vi "Funnel Edit.vi"() -> ()   [LabVIEW 2019]
uses:
  Classes/Settings/Funnel Settings/Funnel Settings.lvclass/Funnel Settings.ctl
  Classes/Settings/ObjectSettings/ObjectSettings.lvclass/ObjectSettings.ctl
  typedefs/Schedule Types/Schedule--Constant.ctl
  Classes/Settings/Setting Database/Setting Database.lvclass
  Classes/Settings/Funnel Settings/Funnel Settings.lvclass
  C:/Users/Albro/Documents/GitHub/AFM-Lithography/lvsrc/Classes/Settings/ObjectSettings/ObjectSettings.lvclass
  Classes/Settings/Setting Database/Typedefs/PrivateEvents--Setting Database.SetDefaultFunnel.ctl
  Classes/Settings/Setting Database/Typedefs/PrivateEvents--Setting Database.CopyActiveFunnelToAll.ctl
  <vilib>/JKI/JKI SMO/SMO/SMO.lvclass
  Classes/Settings/Funnel Settings/Accessors/Write Bottom Segments.vi
  Classes/Settings/ObjectSettings/Accessors/Write Resistance.vi
  Classes/Settings/ObjectSettings/Accessors/Read Speed Settings.vi
  Classes/Settings/ObjectSettings/Accessors/Read Voltage Settings.vi
  Classes/Settings/ObjectSettings/Accessors/Write Enabled.vi
  Classes/Settings/ObjectSettings/Accessors/Write Voltage Schedule.vi
  Classes/Settings/ObjectSettings/Accessors/Write Speed Schedule.vi
  Classes/Settings/ObjectSettings/Accessors/Write Direction.vi
  Classes/Settings/Funnel Settings/Accessors/Write Smooth Segments.vi
  Classes/Settings/ObjectSettings/Accessors/Read Enabled.vi
  Classes/Settings/ObjectSettings/Accessors/Read Direction.vi
  Classes/Settings/Funnel Settings/Accessors/Read Smooth Segments.vi
  Classes/Settings/Funnel Settings/Accessors/Read Bottom Segments.vi
  Classes/Settings/ObjectSettings/Accessors/Read Speed Schedule.vi
  Classes/Settings/ObjectSettings/Accessors/Read Voltage Schedule.vi
  Classes/Settings/ObjectSettings/Accessors/Read Resistance.vi
  Classes/Settings/ObjectSettings/ObjectSettings.lvclass
panel:
  in  "Save Default":bool
  out "resources found?":bool
  in  "Speed Settings":bool
  in  "Voltage Settings":bool
  in  "Smooth Segments":dbl caption="Numeric 2"
  in  "Set Resistance":T1(ring) caption="Enum"
  in  "Copy to All":bool
  in  "Bottom Segments":dbl caption="Numeric 2"
  in  "Voltage (V)":dbl caption="Numeric 2"
  in  "Speed (um/s)":dbl caption="Numeric 2"
  in  "Voltage Schedule":u16(ring) caption="Ring" items=["Constant", "Ramp", "Fn. Generator", "Formula"]
  in  "Speed Schedule":u16(ring) caption="Ring" items=["Constant", "Ramp", "Fn. Generator", "Formula"]
  in  "Direction":u16(ring) caption="Ring" items=["Forward", "Backward"]
  in  "Enabled?":bool=TRUE
  in  "Index":i32=8
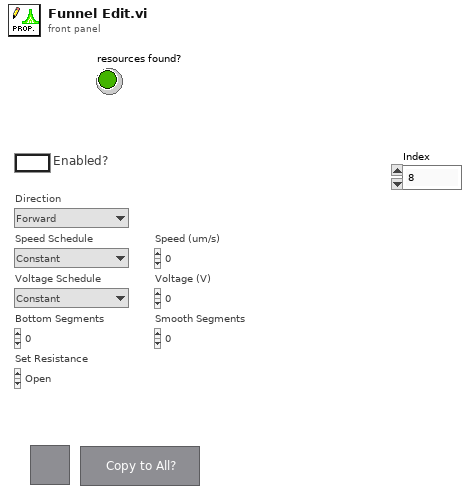
[diagram p1: front panel]
types:
  T1 = enum16{"Open", "Discharge Tip", "0 ohm", "100 kohm", "10 Mohm", "1 Gohm"}
  T2 = typedef "Schedule--Constant.ctl" = cluster{"Value":dbl}
  T3 = enum32{"invalid app kind", "Development System", "Run Time System", "Student Edition", "Embedded LabVIEW", "Evaluation", "Custom"}
  T4 = enum8{"Enabled", "Disabled", "Disabled and Grayed Out"}
  T5 = enum32{"Invalid", "Standard", "Closed", "Hidden", "Minimized", "Maximized"}
  T6 = typedef "Setting Database.lvclass/PrivateEvents--Setting Database.SetDefaultFunnel.ctl" = bool
  T7 = typedef "Setting Database.lvclass/PrivateEvents--Setting Database.CopyActiveFunnelToAll.ctl" = bool
  T8 = typedef "Setting Database.lvclass/PublicEvents--Setting Database.NewActiveFunnel.ctl" = refnum<class "Funnel Settings.lvclass">
  T9 = cluster{"Core":cluster{"Current VI Reference":refnum<vi>, "Close Panel on Exit?":bool}, "SettingDB":refnum<class "Setting Database.lvclass">, "Funnel Settings":refnum<class "Funnel Settings.lvclass">}
  T10 = cluster{"Current VI Reference":refnum<vi>, "Close Panel on Exit?":bool}
  T11 = typedef "Setting Database.lvclass/PublicEvents--Cluster.ctl" = cluster{"NewActivePath":refnum<user-event>, "PathsUpdated":refnum<user-event>, "RectanglesUpdated":refnum<user-event>, "NewActiveRectangle":refnum<user-event>, "NewActiveFunnel":refnum<user-event>, "FunnelsUpdated":refnum<user-event>, "NewActiveDot":refnum<user-event>, "DotsUpdated":refnum<user-event>}
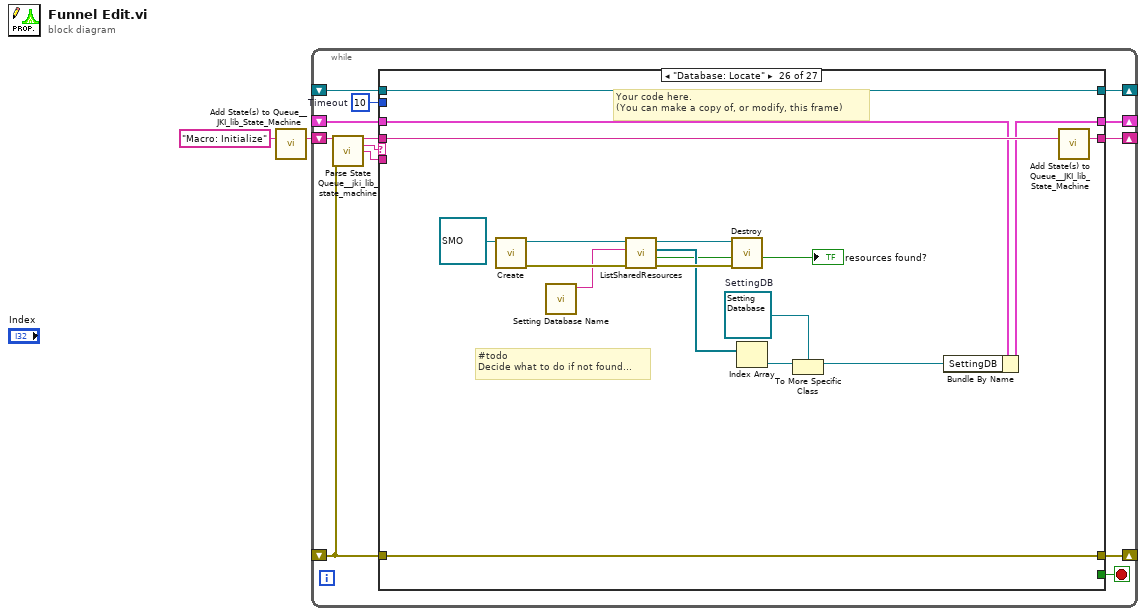
[diagram p0: block diagram]
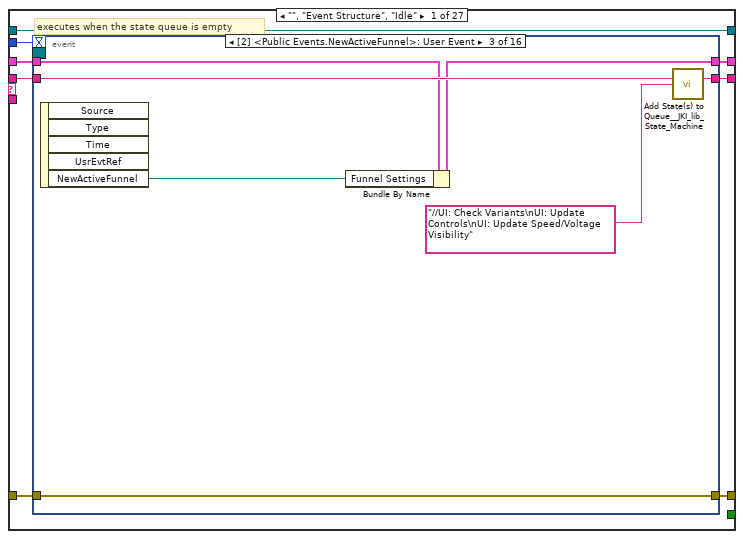
[diagram p2: hidden frame]
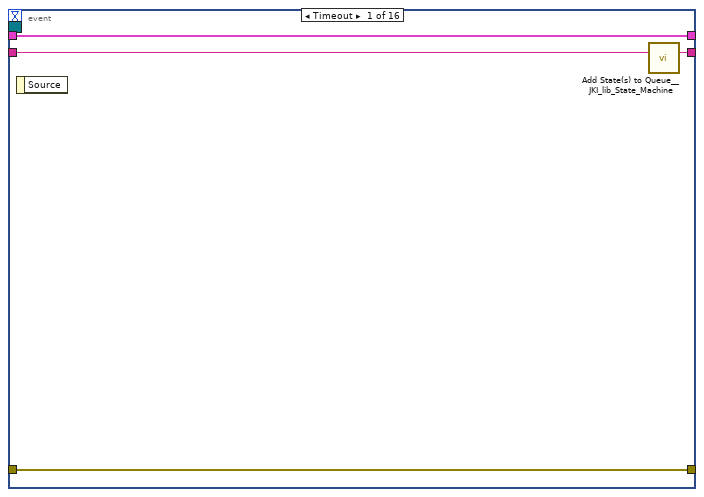
[diagram p3: hidden frame]
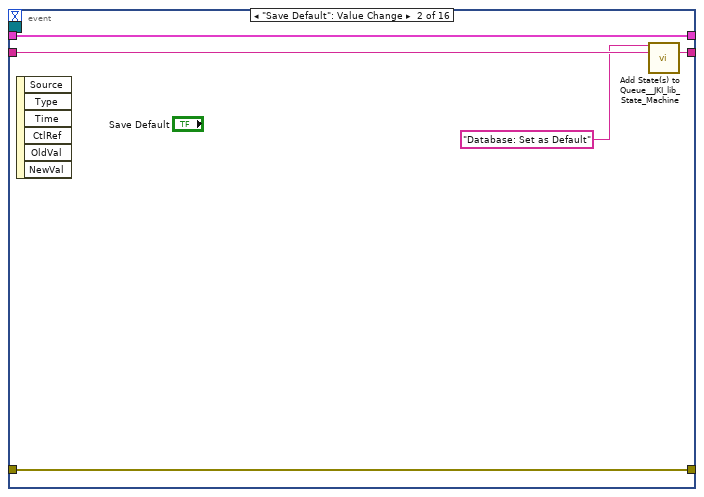
[diagram p4: hidden frame]
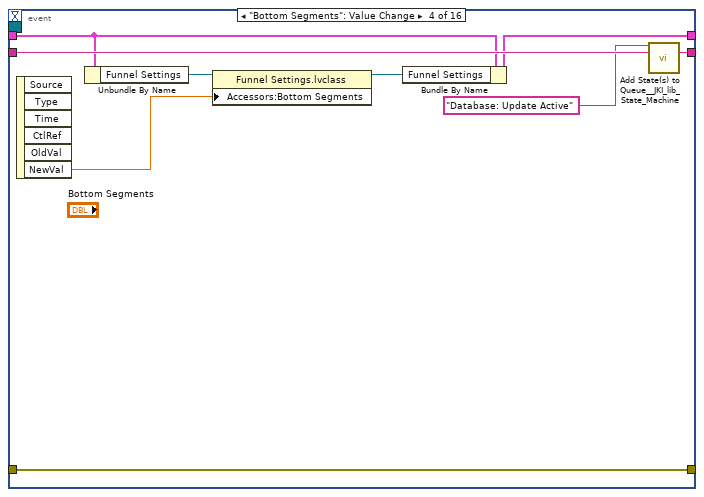
[diagram p5: hidden frame]
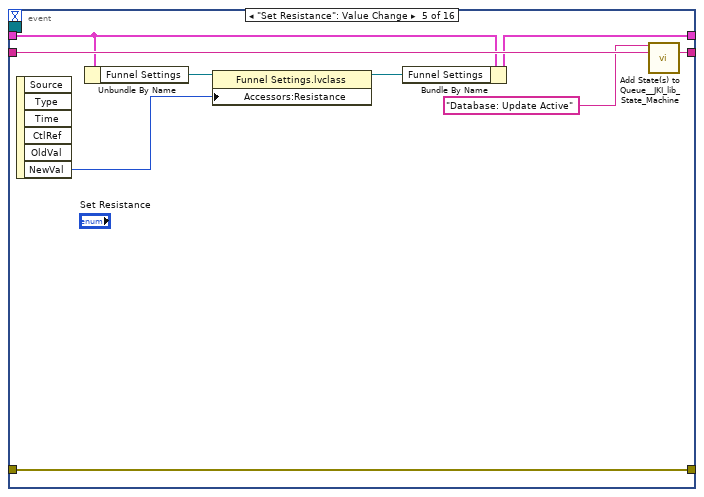
[diagram p6: hidden frame]
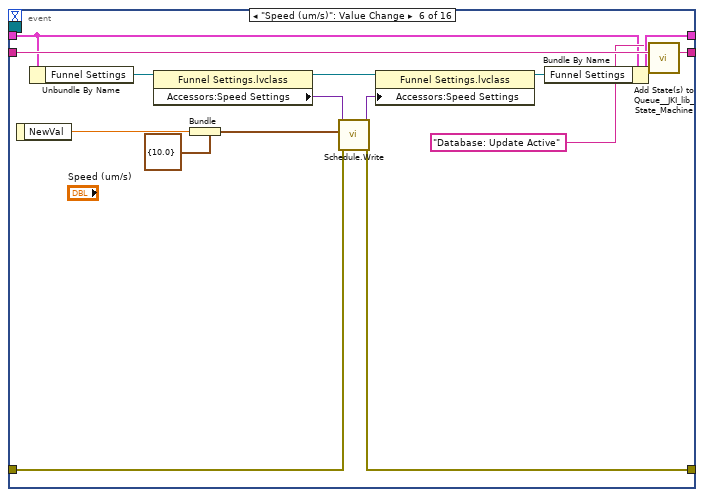
[diagram p7: hidden frame]
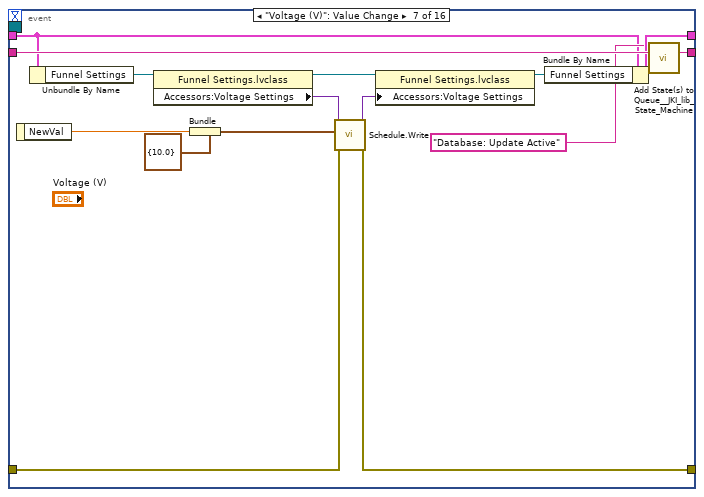
[diagram p8: hidden frame]
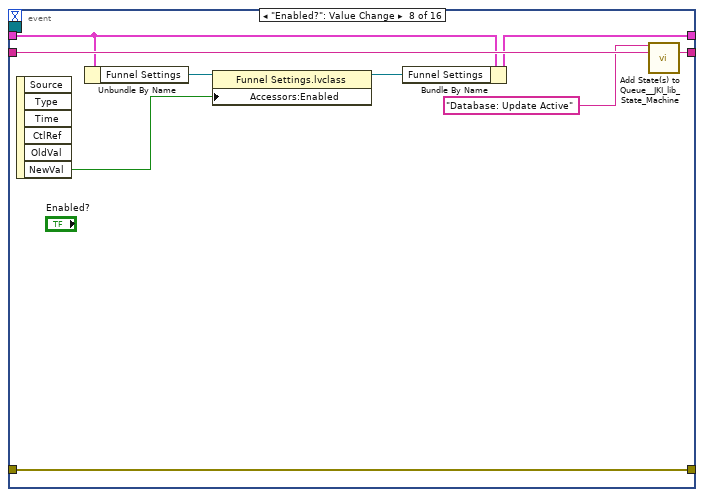
[diagram p9: hidden frame]
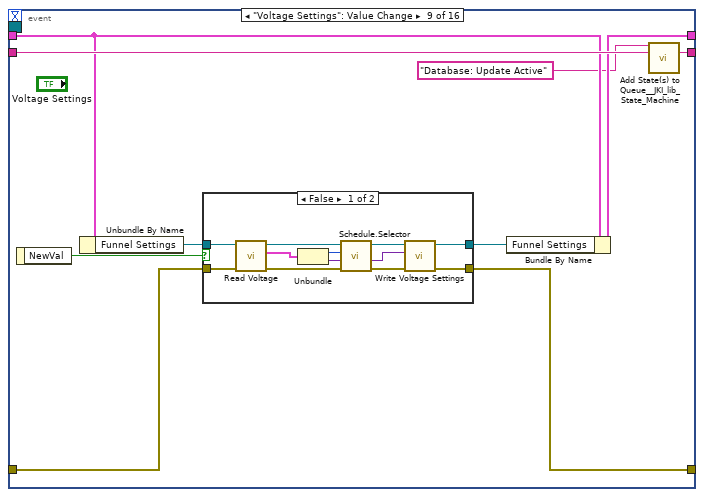
[diagram p10: hidden frame]
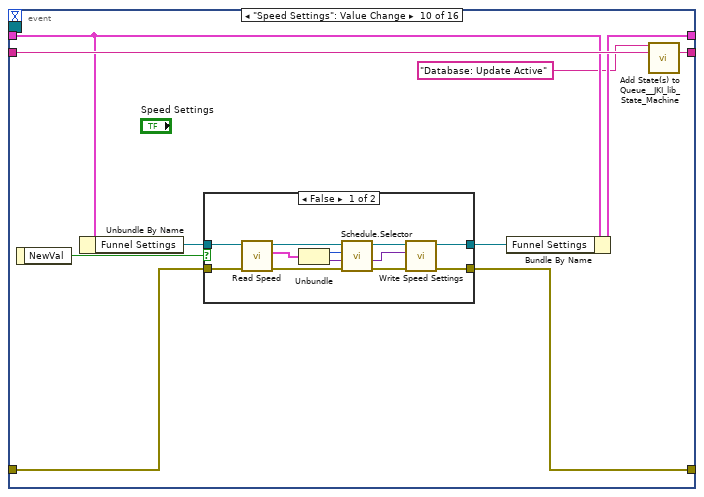
[diagram p12: hidden frame]
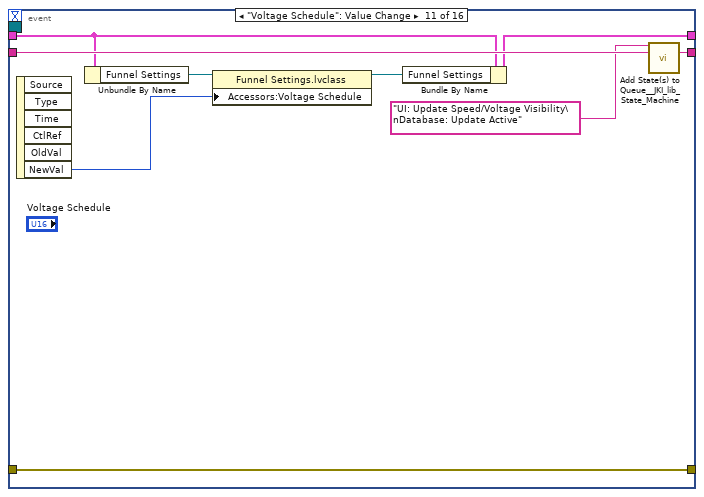
[diagram p14: hidden frame]
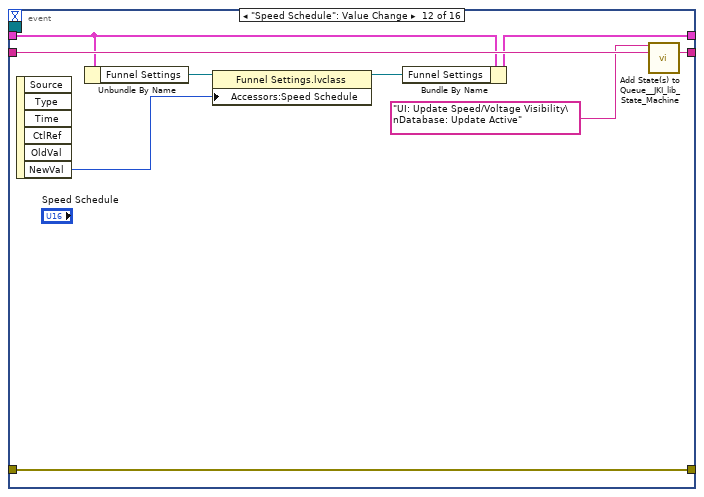
[diagram p15: hidden frame]
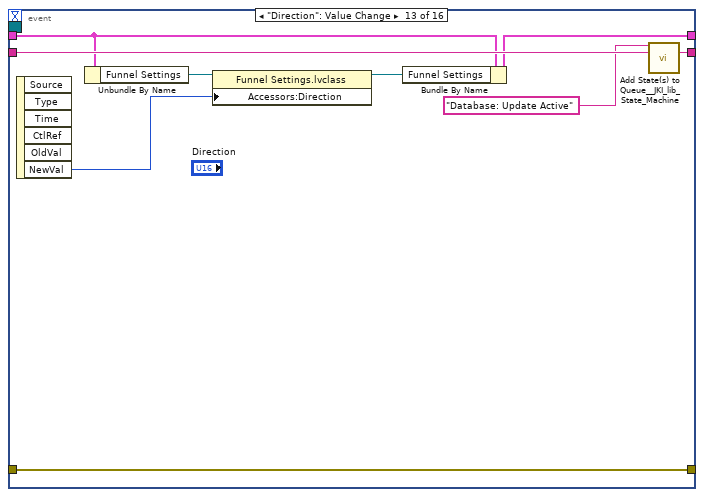
[diagram p16: hidden frame]
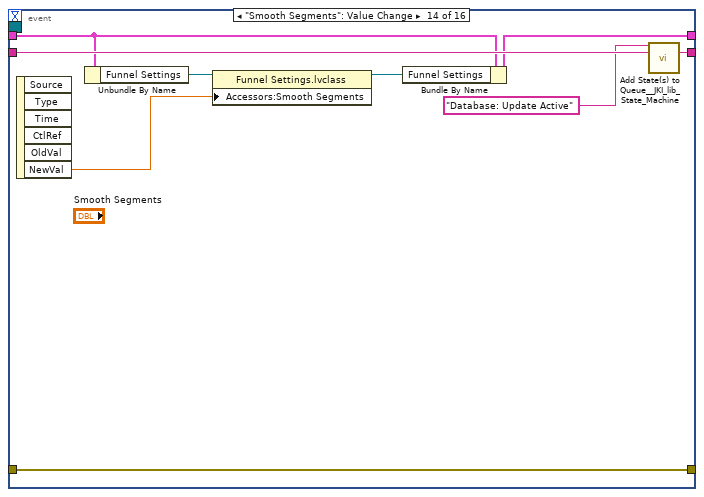
[diagram p17: hidden frame]
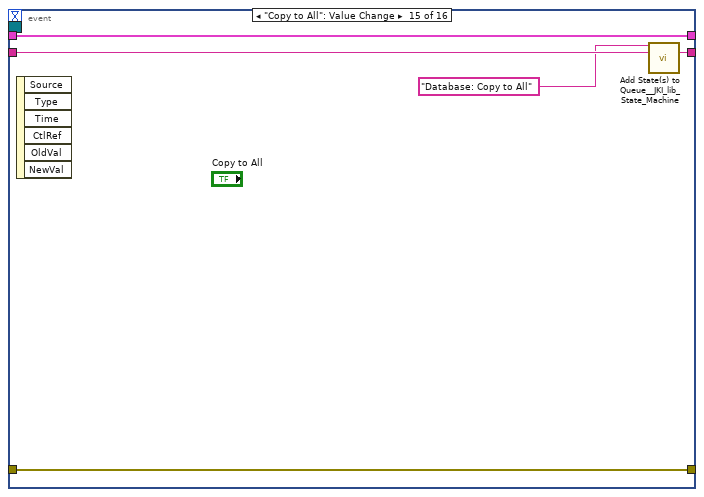
[diagram p18: hidden frame]
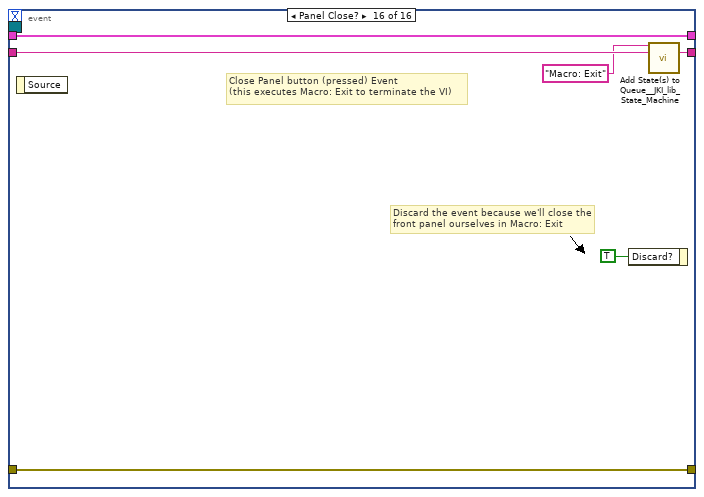
[diagram p19: hidden frame]
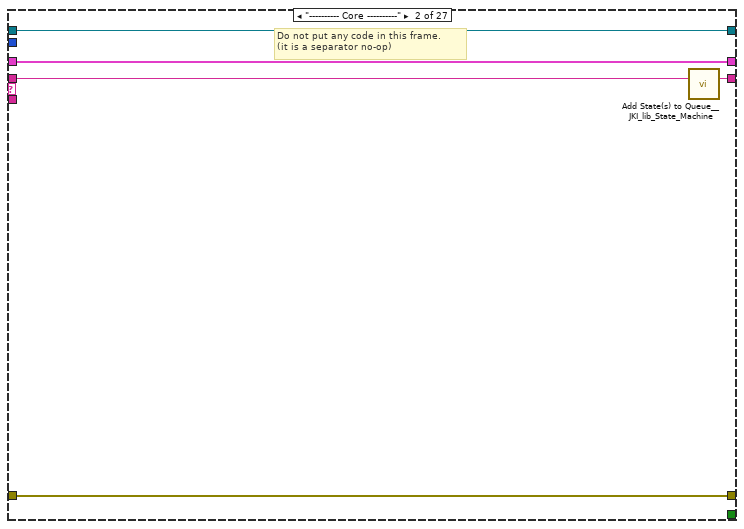
[diagram p20: hidden frame]
diagram:
  n1 = call <vilib>:"Add State(s) to Queue__JKI_lib_State_Machine.vi"("State(s) in (\"\")"="Macro: Initialize") -> ("States Out"=w2:string)  [unwired: 14 in]
  n2 = while "JKI - String-Based Queued State Machine (Basic) v1.0" {
    shift-right: [w8] -> _
    shift-left: _ -> [w7]
    shift-right: [w11] -> _
    shift-left: _ -> [w5]
    shift-right: [w10] -> _
    shift-left: w2 -> [w12]
    shift-right: [w4] -> _
    shift-left: _ -> [w3]
    stop <- w9 stop-if-true
    w6 = 10  # Timeout
    n3 = call <vilib>:"Parse State Queue__jki_lib_state_machine.vi"("State Queue"=w12, "Error In (no error)"=w5) -> ("Remaining States"=w14:string, "Current State"=w15:string, "Arguments"=w13:string)  [unwired: 11 in]
    n4 = case shown="\"Database: Locate\"" w15 {
      selector: w15 -> [_ _ w202 _ _ _ _ _ _ _ _ _ _ _ _ _ _ _ _ _ _ _ _ _ _ _ _]
      tunnel: w14 -> [w23 w196 w200 w221 w228 w234 w239 w247 w254 w259 w269 w275 w280 w288 w312 w327 w334 w353 w365 w392 w398 w409 w414 w424 w434 w451 w461]
      tunnel: w13 -> [_ _ _ _ _ _ _ _ _ _ _ _ _ _ _ _ w330 _ w360 _ _ _ _ _ _ _ _]
      tunnel: w7 -> [w21 w193 w201 w214 w223 w230 w236 _ w251 w256 w265 w273 w277 w286 w306 w319 w329 w351 w359 w389 w394 w400 w411 w416 w430 w438 w457]
      tunnel: [w20 w194 w205 w219 errorcluster {"status"=FALSE, "code"=0, "source"=""} ("error out") w232 w237 w243 w249 w257 w264 w270 w278 w282 w310 w324 w331 w340 w362 w390 w396 w407 w412 w419 w426 w449 w454] -> w11
      tunnel: w5 -> [w19 w194 w204 w219 w225 w232 w237 w243 w250 w257 w263 w271 w278 w281 w310 w323 w332 w350 w363 w390 w396 w407 w412 w418 w427 w449 w453]
      tunnel: [w22 w195 w203 w220 w227 w233 w238 w246 w253 w258 w268 w274 w279 w287 w311 w326 w333 w352 w364 w391 w397 w408 w413 w423 w433 w450 w460] -> w10
      tunnel: [_ _ _ _ _ TRUE _ _ _ _ _ _ _ _ _ _ _ _ _ _ _ _ _ _ _ _ _] -> w9
      tunnel: [w18 w193 w201 w213 w223 w230 w236 w245 w251 w256 w265 w273 w277 w286 w306 w320 w329 w351 w359 w389 w394 w400 w411 w417 w431 w439 w458] -> w8
      tunnel: w6 -> [w17 _ _ _ _ _ _ _ _ _ _ _ _ _ _ _ _ _ _ _ _ _ _ _ _ _ _]
      tunnel: [w16 w192 w197 w209 w222 w229 w235 w241 w248 w255 w267 w272 w276 w285 w307 w322 w328 w339 w358 w388 w393 w399 w410 w422 w432 w436 w459] -> w4
      tunnel: w3 -> [w16 w192 w197 w209 w222 w229 w235 w241 w248 w255 _ w272 w276 w285 w307 w322 w328 w339 w358 w388 w393 w399 w410 w422 w432 w436 w459]
      frame "", "Event Structure", "Idle" {
        # "executes when the state queue is empty"
        n5 = event shown="[2] <Public Events.NewActiveFunnel>: User Event" {
          selector: w16 -> [_ _ _ _ _ _ _ _ _ _ _ _ _ _ _ _]
          dyn-events: _ -> [_ _ _ _ _ _ _ _ _ _ _ _ _ _ _ _]
          timeout: w17 -> [_ _ _ _ _ _ _ _ _ _ _ _ _ _ _ _]
          tunnel: w23 -> [w27 w32 w39 w48 w57 w72 w87 w96 w106 w130 w153 w162 w171 w180 w185 w191]
          tunnel: [w26 w31 w38 w47 w56 w71 w86 w95 w105 w129 w152 w161 w170 w179 w184 w190] -> w22
          tunnel: w21 -> [w24 w29 w34 w44 w53 w65 w80 w92 w103 w127 w149 w158 w167 w176 w183 w188]
          tunnel: [w25 w30 w37 w46 w55 w58 w73 w94 w99 w122 w151 w160 w169 w178 w182 w189] -> w20
          tunnel: w19 -> [w25 w30 w37 w46 w55 w59 w74 w94 w98 w123 w151 w160 w169 w178 w182 w189]
          tunnel: [w24 w29 w35 w45 w54 w70 w85 w93 w104 w128 w150 w159 w168 w177 w183 w188] -> w18
          event Timeout {
            n6 = event-data() -> ()  [unwired: 1 in, 1 out]
            n7 = call <vilib>:"Add State(s) to Queue__JKI_lib_State_Machine.vi"("State(s) in (\"\")"=w27) -> ("States Out"=w26:string)  [unwired: 14 in]
          }
          event "Save Default": Value Change {
            n8 = event-data() -> ()  [unwired: 1 in, 6 out]
            n9 = call <vilib>:"Add State(s) to Queue__JKI_lib_State_Machine.vi"("State(s) in Front (\"\")"="Database: Set as Default", "State(s) in (\"\")"=w32) -> ("States Out"=w31:string)  [unwired: 13 in]
          }
          event User Event {
            n10 = event-data() -> ("NewActiveFunnel"=w33:T8)  [unwired: 1 in, 4 out]
            n11 = Bundle By Name(cluster=w34, "Funnel Settings"=w33) -> (w35:T9)
            n12 = call <vilib>:"Add State(s) to Queue__JKI_lib_State_Machine.vi"("State(s) in (\"\")"=w39, "State(s) at Back (\"\")"="//UI: Check Variants\nUI: Update Controls\nUI: Update Speed/Voltage Visibility") -> ("States Out"=w38:string)  [unwired: 13 in]
          }
          event "Bottom Segments": Value Change {
            n13 = event-data() -> ("NewVal"=w41:dbl)  [unwired: 1 in, 5 out]
            n14 = Unbundle By Name(w44) -> ("Funnel Settings"=w43:refnum<class "Funnel Settings.lvclass">)
            n15 = property class="Funnel Settings.lvclass"(reference=w43, "Accessors:Bottom Segments"=w41) -> (reference out=w42:refnum<class "Funnel Settings.lvclass">)  [unwired: 1 in, 1 out]
            n16 = Bundle By Name(cluster=w44, "Funnel Settings"=w42) -> (w45:T9)
            n17 = call <vilib>:"Add State(s) to Queue__JKI_lib_State_Machine.vi"("State(s) in Front (\"\")"="Database: Update Active", "State(s) in (\"\")"=w48) -> ("States Out"=w47:string)  [unwired: 13 in]
          }
          event "Set Resistance": Value Change {
            n18 = event-data() -> ("NewVal"=w50:T1)  [unwired: 1 in, 5 out]
            n19 = Unbundle By Name(w53) -> ("Funnel Settings"=w52:refnum<class "Funnel Settings.lvclass">)
            n20 = property class="Funnel Settings.lvclass"(reference=w52, "Accessors:Resistance"=w50) -> (reference out=w51:refnum<class "Funnel Settings.lvclass">)  [unwired: 1 in, 1 out]
            n21 = Bundle By Name(cluster=w53, "Funnel Settings"=w51) -> (w54:T9)
            n22 = call <vilib>:"Add State(s) to Queue__JKI_lib_State_Machine.vi"("State(s) in Front (\"\")"="Database: Update Active", "State(s) in (\"\")"=w57) -> ("States Out"=w56:string)  [unwired: 13 in]
          }
          event "Speed (um/s)": Value Change {
            n23 = event-data() -> ("NewVal"=w63:dbl)  [unwired: 1 in]
            n24 = Unbundle By Name(w65) -> ("Funnel Settings"=w69:refnum<class "Funnel Settings.lvclass">)
            n25 = property class="Funnel Settings.lvclass"(reference=w69) -> (reference out=w68:refnum<class "Funnel Settings.lvclass">, "Accessors:Speed Settings"=w62:variant)  [unwired: 1 in, 1 out]
            n26 = Bundle(cluster=T2 {"Value"=10.0} ("Constant"), "Value"=w63) -> (w60:T2)
            n27 = call "Schedule.Write.vi"("error in (no error)"=w59, "Data to Write"=w60, "LUT In"=w62) -> ("error out"=w58:errorcluster, "LUT Out"=w61:variant)  [unwired: 7 in]
            n28 = property class="Funnel Settings.lvclass"(reference=w68, "Accessors:Speed Settings"=w61) -> (reference out=w66:refnum<class "Funnel Settings.lvclass">)  [unwired: 1 in, 1 out]
            n29 = Bundle By Name(cluster=w65, "Funnel Settings"=w66) -> (w70:T9)
            n30 = call <vilib>:"Add State(s) to Queue__JKI_lib_State_Machine.vi"("State(s) in Front (\"\")"="Database: Update Active", "State(s) in (\"\")"=w72) -> ("States Out"=w71:string)  [unwired: 13 in]
          }
          event "Voltage (V)": Value Change {
            n31 = event-data() -> ("NewVal"=w78:dbl)  [unwired: 1 in]
            n32 = Unbundle By Name(w80) -> ("Funnel Settings"=w84:refnum<class "Funnel Settings.lvclass">)
            n33 = property class="Funnel Settings.lvclass"(reference=w84) -> (reference out=w83:refnum<class "Funnel Settings.lvclass">, "Accessors:Voltage Settings"=w77:variant)  [unwired: 1 in, 1 out]
            n34 = Bundle(cluster=T2 {"Value"=10.0} ("Constant"), "Value"=w78) -> (w75:T2)
            n35 = call "Schedule.Write.vi"("error in (no error)"=w74, "Data to Write"=w75, "LUT In"=w77) -> ("error out"=w73:errorcluster, "LUT Out"=w76:variant)  [unwired: 7 in]
            n36 = property class="Funnel Settings.lvclass"(reference=w83, "Accessors:Voltage Settings"=w76) -> (reference out=w81:refnum<class "Funnel Settings.lvclass">)  [unwired: 1 in, 1 out]
            n37 = Bundle By Name(cluster=w80, "Funnel Settings"=w81) -> (w85:T9)
            n38 = call <vilib>:"Add State(s) to Queue__JKI_lib_State_Machine.vi"("State(s) in Front (\"\")"="Database: Update Active", "State(s) in (\"\")"=w87) -> ("States Out"=w86:string)  [unwired: 13 in]
          }
          event "Enabled?": Value Change {
            n39 = event-data() -> ("NewVal"=w89:bool)  [unwired: 1 in, 5 out]
            n40 = Unbundle By Name(w92) -> ("Funnel Settings"=w91:refnum<class "Funnel Settings.lvclass">)
            n41 = property class="Funnel Settings.lvclass"(reference=w91, "Accessors:Enabled"=w89) -> (reference out=w90:refnum<class "Funnel Settings.lvclass">)  [unwired: 1 in, 1 out]
            n42 = Bundle By Name(cluster=w92, "Funnel Settings"=w90) -> (w93:T9)
            n43 = call <vilib>:"Add State(s) to Queue__JKI_lib_State_Machine.vi"("State(s) in Front (\"\")"="Database: Update Active", "State(s) in (\"\")"=w96) -> ("States Out"=w95:string)  [unwired: 13 in]
          }
          event "Voltage Settings": Value Change {
            n44 = event-data() -> ("NewVal"=w97:bool)  [unwired: 1 in]
            n45 = Unbundle By Name(w103) -> ("Funnel Settings"=w101:refnum<class "Funnel Settings.lvclass">)
            n46 = case shown="False" w97 {
              tunnel: w101 -> [w118 w120]
              tunnel: [w110 w120] -> w100
              tunnel: w98 -> [w117 w119]
              tunnel: [w107 w119] -> w99
              frame False {
                n47 = call "Read Voltage.vi"("error in (no error)"=w117, "ObjectSettings in"=w118) -> ("error out"=w115:errorcluster, "Voltage"=w114:cluster{"Schedule":u16, "Settings":variant}, "ObjectSettings out"=w116:refnum<class "Funnel Settings.lvclass">)  [unwired: 7 in]
                n48 = Unbundle(w114) -> ("Schedule"=w113:u16, "Settings"=w112:variant)
                n49 = call-dynamic "Schedule.Selector.vi"("error in (no error)"=w115, "Settings In"=w112, "Schedule"=w113, "ObjectSettings in"=w116) -> ("error out"=w109:errorcluster, "Settings Out"=w108:variant, "ObjectSettings out"=w111:refnum<class "Funnel Settings.lvclass">)  [unwired: 5 in]
                n50 = call "Write Voltage Settings.vi"("error in (no error)"=w109, "Settings"=w108, "ObjectSettings in"=w111) -> ("error out"=w107:errorcluster, "ObjectSettings out"=w110:refnum<class "Funnel Settings.lvclass">)  [unwired: 7 in]
              }
              frame True {
              }
            }
            n51 = Bundle By Name(cluster=w103, "Funnel Settings"=w100) -> (w104:T9)
            n52 = call <vilib>:"Add State(s) to Queue__JKI_lib_State_Machine.vi"("State(s) in Front (\"\")"="Database: Update Active", "State(s) in (\"\")"=w106) -> ("States Out"=w105:string)  [unwired: 13 in]
          }
          event "Speed Settings": Value Change {
            n53 = event-data() -> ("NewVal"=w124:bool)  [unwired: 1 in]
            n54 = Unbundle By Name(w127) -> ("Funnel Settings"=w125:refnum<class "Funnel Settings.lvclass">)
            n55 = case shown="False" w124 {
              tunnel: w125 -> [w140 w144]
              tunnel: [w134 w144] -> w121
              tunnel: w123 -> [w138 w143]
              tunnel: [w133 w143] -> w122
              frame False {
                n56 = call "Read Speed.vi"("error in (no error)"=w138, "ObjectSettings in"=w140) -> ("error out"=w137:errorcluster, "Speed"=w136:cluster{"Schedule":u16, "Settings":variant}, "ObjectSettings out"=w139:refnum<class "Funnel Settings.lvclass">)  [unwired: 7 in]
                n57 = Unbundle(w136) -> ("Schedule"=w142:u16, "Settings"=w141:variant)
                n58 = call-dynamic "Schedule.Selector.vi"("error in (no error)"=w137, "Settings In"=w141, "Schedule"=w142, "ObjectSettings in"=w139) -> ("error out"=w132:errorcluster, "Settings Out"=w131:variant, "ObjectSettings out"=w135:refnum<class "Funnel Settings.lvclass">)  [unwired: 5 in]
                n59 = call "Write Speed Settings.vi"("error in (no error)"=w132, "Settings"=w131, "ObjectSettings in"=w135) -> ("error out"=w133:errorcluster, "ObjectSettings out"=w134:refnum<class "Funnel Settings.lvclass">)  [unwired: 7 in]
              }
              frame True {
              }
            }
            n60 = Bundle By Name(cluster=w127, "Funnel Settings"=w121) -> (w128:T9)
            n61 = call <vilib>:"Add State(s) to Queue__JKI_lib_State_Machine.vi"("State(s) in Front (\"\")"="Database: Update Active", "State(s) in (\"\")"=w130) -> ("States Out"=w129:string)  [unwired: 13 in]
          }
          event "Voltage Schedule": Value Change {
            n62 = event-data() -> ("NewVal"=w146:u16)  [unwired: 1 in, 5 out]
            n63 = Unbundle By Name(w149) -> ("Funnel Settings"=w148:refnum<class "Funnel Settings.lvclass">)
            n64 = property class="Funnel Settings.lvclass"(reference=w148, "Accessors:Voltage Schedule"=w146) -> (reference out=w147:refnum<class "Funnel Settings.lvclass">)  [unwired: 1 in, 1 out]
            n65 = Bundle By Name(cluster=w149, "Funnel Settings"=w147) -> (w150:T9)
            n66 = call <vilib>:"Add State(s) to Queue__JKI_lib_State_Machine.vi"("State(s) in Front (\"\")"="UI: Update Speed/Voltage Visibility\nDatabase: Update Active", "State(s) in (\"\")"=w153) -> ("States Out"=w152:string)  [unwired: 13 in]
          }
          event "Speed Schedule": Value Change {
            n67 = event-data() -> ("NewVal"=w155:u16)  [unwired: 1 in, 5 out]
            n68 = Unbundle By Name(w158) -> ("Funnel Settings"=w157:refnum<class "Funnel Settings.lvclass">)
            n69 = property class="Funnel Settings.lvclass"(reference=w157, "Accessors:Speed Schedule"=w155) -> (reference out=w156:refnum<class "Funnel Settings.lvclass">)  [unwired: 1 in, 1 out]
            n70 = Bundle By Name(cluster=w158, "Funnel Settings"=w156) -> (w159:T9)
            n71 = call <vilib>:"Add State(s) to Queue__JKI_lib_State_Machine.vi"("State(s) in Front (\"\")"="UI: Update Speed/Voltage Visibility\nDatabase: Update Active", "State(s) in (\"\")"=w162) -> ("States Out"=w161:string)  [unwired: 13 in]
          }
          event "Direction": Value Change {
            n72 = event-data() -> ("NewVal"=w164:u16)  [unwired: 1 in, 5 out]
            n73 = Unbundle By Name(w167) -> ("Funnel Settings"=w166:refnum<class "Funnel Settings.lvclass">)
            n74 = property class="Funnel Settings.lvclass"(reference=w166, "Accessors:Direction"=w164) -> (reference out=w165:refnum<class "Funnel Settings.lvclass">)  [unwired: 1 in, 1 out]
            n75 = Bundle By Name(cluster=w167, "Funnel Settings"=w165) -> (w168:T9)
            n76 = call <vilib>:"Add State(s) to Queue__JKI_lib_State_Machine.vi"("State(s) in Front (\"\")"="Database: Update Active", "State(s) in (\"\")"=w171) -> ("States Out"=w170:string)  [unwired: 13 in]
          }
          event "Smooth Segments": Value Change {
            n77 = event-data() -> ("NewVal"=w173:dbl)  [unwired: 1 in, 5 out]
            n78 = Unbundle By Name(w176) -> ("Funnel Settings"=w175:refnum<class "Funnel Settings.lvclass">)
            n79 = property class="Funnel Settings.lvclass"(reference=w175, "Accessors:Smooth Segments"=w173) -> (reference out=w174:refnum<class "Funnel Settings.lvclass">)  [unwired: 1 in, 1 out]
            n80 = Bundle By Name(cluster=w176, "Funnel Settings"=w174) -> (w177:T9)
            n81 = call <vilib>:"Add State(s) to Queue__JKI_lib_State_Machine.vi"("State(s) in Front (\"\")"="Database: Update Active", "State(s) in (\"\")"=w180) -> ("States Out"=w179:string)  [unwired: 13 in]
          }
          event "Copy to All": Value Change {
            n82 = event-data() -> ()  [unwired: 1 in, 6 out]
            n83 = call <vilib>:"Add State(s) to Queue__JKI_lib_State_Machine.vi"("State(s) in Front (\"\")"="Database: Copy to All", "State(s) in (\"\")"=w185) -> ("States Out"=w184:string)  [unwired: 13 in]
          }
          event Panel Close? {
            # "Discard the event because we'll close the front panel ourselves in Macro: Exit"
            # "Close Panel button (pressed) Event\n(this executes Macro: Exit to terminate the VI)"
            n84 = event-data() -> ()  [unwired: 1 in, 1 out]
            n85 = event-data("Discard?"=TRUE) -> ()  [unwired: 1 in, 1 out]
            n86 = call <vilib>:"Add State(s) to Queue__JKI_lib_State_Machine.vi"("State(s) in Front (\"\")"="Macro: Exit", "State(s) in (\"\")"=w191) -> ("States Out"=w190:string)  [unwired: 13 in]
          }
        }
      }
      frame "---------- Core ----------" {
        # "Do not put any code in this frame.\n(it is a separator no-op)"
        n87 = call <vilib>:"Add State(s) to Queue__JKI_lib_State_Machine.vi"("State(s) in (\"\")"=w196) -> ("States Out"=w195:string)  [unwired: 14 in]
      }
      frame Default {
        w208 = 42 items=["No error", "Argument error", "Memory is full", "Out of zone", "End of file", "File already open", "Generic file I/O error", "File not found", "File permission error", "Disk is full", "Duplicate path", "Too many files open", "System feature not enabled", "Resource file not found", "Cannot add resource", "Resource not found", "Image not found", "Image memory error", "Pen does not exist", "Config type invalid", "Config token not found", "Config parse error", "Config memory error", "Bad external code format", "Bad external code offset", "External code not present", "Null window", "Destroy window error", "Null menu", "Print aborted", "Bad print record", "Print driver error", "Windows error during printing", "Memory error during printing", "Print dialog error", "Generic print error", "Invalid device refnum", "Device not found", "Device parameter error", "Device unit error", "Cannot open device", "Device call aborted", "Generic error", "Cancelled by user", "Object ID too low", "Object ID too high", "Object not in heap", "Unknown heap", "Unknown object (invalid DefProc)", "Unknown object (DefProc not in table)", "Message out of range", "Invalid (null) method", "Unknown message", "Manager call not supported", "Bad address", "Network operation in progress", "Network operation timed out", "Connection is busy", "Network attribute not supported", "Network error", "Address in use", "System out of memory", "Connection aborted", "Connection refused", "Not connected", "Already connected", "Connection closed", "Initialization error (interapplication manager)", "Bad occurrence", "Wait on unbound occurrence handler", "Occurrence queue overflow", "Datalog type conflict", "Unused", "Unrecognized type (interapplication manager)", "Memory corrupt", "Failed to make temporary DLL", "Old CIN version", "Drag socket not found", "Failed to load drop-object", "Failed to register OLE object", "Failed to release OLE object", "Format specifier type mismatch", "Unknown format specifier", "Too few format specifiers", "Too many format specifiers", "Scan failed", "Newer CIN version", "Error converting to variant", "Runtime menu error", "Password tampered", "Variant attribute not found", "Incompatible variant data type", "Event data is not available", "Event Store is not present", "Occurrence is not found", "Event Queue is not created", "Event info is not available", "Refnum passed is NULL", "Error retrieving Class GUID", "Error retrieving CoClass GUID", "Error retrieving TypeLib GUID.", "Bad built application magic bytes.", "Specific driver is different from the specific driver associated with the Logical Name.", "There is no session opened to the class driver.", "Max Error", "MAX - Error with config objects", "MAX - Error loading configuration", "MAX - Group not supported"]
        # "Current State"
        # "Do not delete, rename, or modify this frame.\n(this is used to capture unhandled states and typos)"
        # "Handle mistyped state name (developer tool)"
        n88 = Format Into String(format string="Software Exception: Unhandled State \"%s\"." ("message"), error in=w204, w202) -> (resulting string=w207:string, error out=w206:errorcluster)  [unwired: 1 in]
        n89 = call <vilib>:"Error Cluster From Error Code.vi"("show call chain? (False)"=TRUE, "error in (no error)"=w206, "error message (\"\")"=w207, "error code (0)"=w208) -> ("error out"=w205:errorcluster)  [unwired: 5 in]
        n90 = call <vilib>:"Add State(s) to Queue__JKI_lib_State_Machine.vi"("State(s) in (\"\")"=w200) -> ("States Out"=w203:string)  [unwired: 14 in]
      }
      frame "Initialize Core Data" {
        # "exe?"
        # "If panel starts closed or is an EXE, then close it when we exit"
        # "Do not delete, rename, or modify this frame.\n(this is used to determine panel behavior on exit)"
        n91 = control-ref of="Current VI Reference"() -> (w218:refnum<vi>)
        n92 = property class="VI"() -> ("Front Panel.Open"=w217:bool)  [unwired: 2 in, 2 out]
        n93 = property class="App"() -> ("App.Kind"=w216:T3)  [unwired: 2 in, 2 out]
        n94 = Not(x=w217) -> (.not. x?=w212:bool)
        n95 = Equal?(x=w216, y=T3."Run Time System" ("Application:Kind")) -> (x = y?=w211:bool)
        n96 = Or(x=w212, y=w211) -> (x .or. y?=w215:bool)
        n97 = Bundle By Name(cluster=w214, "Core.Current VI Reference"=w218, "Core.Close Panel on Exit?"=w215) -> (w213:T9)
        n98 = call <vilib>:"Add State(s) to Queue__JKI_lib_State_Machine.vi"("State(s) in (\"\")"=w221) -> ("States Out"=w220:string)  [unwired: 14 in]
      }
      frame "Error Handler" {
        # "Unhandled Error -- Display it"
        # "Handle any errors here.\nYou can also output any states to clean-up after errors occur"
        # "Clear error"
        n99 = call <vilib>:"General Error Handler.vi"("error in (no error)"=w225) -> ()  [unwired: 10 in, 5 out]
        n100 = call <vilib>:"Add State(s) to Queue__JKI_lib_State_Machine.vi"("State(s) in Front (\"\")"="/* Post Error States", "State(s) in (\"\")"=w228) -> ("States Out"=w227:string)  [unwired: 13 in]
      }
      frame "Exit" {
        # "Do not put any code in this frame.\n(No errors that occur here will be handled.)"
        n101 = call <vilib>:"Add State(s) to Queue__JKI_lib_State_Machine.vi"("State(s) in (\"\")"=w234) -> ("States Out"=w233:string)  [unwired: 14 in]
      }
      frame "---------- Data ----------" {
        # "Do not put any code in this frame.\n(It is a separator no-op. You can make a copy of this frame to create a new Data frame)"
        n102 = call <vilib>:"Add State(s) to Queue__JKI_lib_State_Machine.vi"("State(s) in (\"\")"=w239) -> ("States Out"=w238:string)  [unwired: 14 in]
      }
      frame "Data: Initialize" {
        w240 = refnum<class "Funnel Settings.lvclass"> refnum  # Funnel Settings
        w242 = refnum<class "Setting Database.lvclass"> refnum  # SettingDB
        w244 = T10 {"Current VI Reference"=refnum, "Close Panel on Exit?"=FALSE}  # Core
        # "Initialize the shift-register data, here.\n(data names are defined by what you wire into the bundle function)"
        n103 = Bundle("Core"=w244, "SettingDB"=w242, "Funnel Settings"=w240) -> (w245:T9)  [unwired: 1 in]
        n104 = call <vilib>:"Add State(s) to Queue__JKI_lib_State_Machine.vi"("State(s) in (\"\")"=w247) -> ("States Out"=w246:string)  [unwired: 14 in]
      }
      frame "Data: Cleanup" {
        # "Cleanup any data and references, here.\n(this is called automatically, by the Macro: Exit)"
        n105 = Unbundle By Name(w251) -> ("Core.Current VI Reference"=w252:refnum<vi>)
        n106 = Close Reference(reference=w252, error in (no error)=w250) -> (error out=w249:errorcluster)
        n107 = call <vilib>:"Add State(s) to Queue__JKI_lib_State_Machine.vi"("State(s) in (\"\")"=w254) -> ("States Out"=w253:string)  [unwired: 14 in]
      }
      frame "---------- Events ----------" {
        # "Do not put any code in this frame.\n(It is a separator no-op. You can make a copy of this frame to create a new UI frame)"
        n108 = call <vilib>:"Add State(s) to Queue__JKI_lib_State_Machine.vi"("State(s) in (\"\")"=w259) -> ("States Out"=w258:string)  [unwired: 14 in]
      }
      frame "Events: Register" {
        # "Do not put any code in this frame.\n(It is a separator no-op. You can make a copy of this frame to create a new UI frame)"
        n109 = Unbundle By Name(w265) -> ("SettingDB"=w261:refnum<class "Setting Database.lvclass">)
        n110 = call "Setting Database.GetPublicEvents.vi"("Setting Database"=w261) -> ("error out"=w262:errorcluster, "Public Events"=w260:T11)  [unwired: 8 in, 1 out]
        n111 = register-events(w260) -> (reference out=w267:refnum<event-registration>, error out=w266:errorcluster)  [unwired: 2 in]
        n112 = Merge Errors(w263, w266, w262) -> (w264:errorcluster)
        n113 = call <vilib>:"Add State(s) to Queue__JKI_lib_State_Machine.vi"("State(s) in (\"\")"=w269) -> ("States Out"=w268:string)  [unwired: 14 in]
      }
      frame "Events: Unregister" {
        # "Do not put any code in this frame.\n(It is a separator no-op. You can make a copy of this frame to create a new UI frame)"
        n114 = Unregister For Events(event registration refnum=w272, error in=w271) -> (error out=w270:errorcluster)
        n115 = call <vilib>:"Add State(s) to Queue__JKI_lib_State_Machine.vi"("State(s) in (\"\")"=w275) -> ("States Out"=w274:string)  [unwired: 14 in]
      }
      frame "---------- UI ----------" {
        # "Do not put any code in this frame.\n(It is a separator no-op. You can make a copy of this frame to create a new UI frame)"
        n116 = call <vilib>:"Add State(s) to Queue__JKI_lib_State_Machine.vi"("State(s) in (\"\")"=w280) -> ("States Out"=w279:string)  [unwired: 14 in]
      }
      frame "UI: Initialize" {
        # "Initialize the User Interface, here.\n(this is called automatically, by the Macro: Init)"
        n117 = control-ref of="Speed Schedule"() -> (w284:refnum<vi>)
        n118 = property class="Ring (strict)"(reference=w284, error in=w281, "DisabledEnum"=T4."Disabled and Grayed Out" ("Disabled")) -> (error out=w282:errorcluster)  [unwired: 1 out]
        n119 = call <vilib>:"Add State(s) to Queue__JKI_lib_State_Machine.vi"("State(s) in (\"\")"=w288) -> ("States Out"=w287:string)  [unwired: 14 in]
      }
      frame "UI: Update Controls" {
        w293 = T2 {"Value"=10.0} ("Constant")
        # "Using Variant Attr. For Settings"
        n120 = Unbundle By Name(w306) -> ("Funnel Settings"=w299:refnum<class "Funnel Settings.lvclass">)
        n121 = property class="Funnel Settings.lvclass"(reference=w299) -> ("Accessors:Enabled"=w305:bool, "Accessors:Direction"=w304:u16, "Accessors:Smooth Segments"=w303:dbl, "Accessors:Bottom Segments"=w302:dbl, "Accessors:Speed Schedule"=w301:u16, "Accessors:Voltage Schedule"=w300:u16, "Accessors:Resistance"=w298:T1, "Accessors:Speed Settings"=w291:variant, "Accessors:Voltage Settings"=w289:variant)  [unwired: 1 in, 2 out]
        n122 = local write "Direction"(w304) -> ()
        n123 = local write "Bottom Segments"(w302) -> ()
        n124 = local write "Voltage Schedule"(w300) -> ()
        n125 = call "Schedule.CheckVariantAttributes.vi"("Variant In"=w291) -> ("Variant Out"=w292:variant)  [unwired: 9 in, 1 out]
        n126 = call "Schedule.CheckVariantAttributes.vi"("Variant In"=w289) -> ("Variant Out"=w290:variant)  [unwired: 9 in, 1 out]
        n127 = call "Schedule.Read.vi"("Data to Read"=w293, "LUT In"=w292) -> ("Data Out"=w297:variant)  [unwired: 7 in, 2 out]
        n128 = call "Schedule.Read.vi"("Data to Read"=w293, "LUT In"=w290) -> ("Data Out"=w296:variant)  [unwired: 7 in, 2 out]
        n129 = local write "Enabled?"(w305) -> ()
        n130 = local write "Smooth Segments"(w303) -> ()
        n131 = local write "Speed Schedule"(w301) -> ()
        n132 = local write "Set Resistance"(w298) -> ()
        n133 = Variant To Data(type=w293, Variant=w297) -> (data=w294:T2)  [unwired: 1 in, 1 out]
        n134 = Variant To Data(type=w293, Variant=w296) -> (data=w295:T2)  [unwired: 1 in, 1 out]
        n135 = Unbundle(w295) -> ("Value"=w308:dbl)
        n136 = Unbundle(w294) -> ("Value"=w309:dbl)
        n137 = local write "Speed (um/s)"(w309) -> ()
        n138 = local write "Voltage (V)"(w308) -> ()
        n139 = call <vilib>:"Add State(s) to Queue__JKI_lib_State_Machine.vi"("State(s) in (\"\")"=w312) -> ("States Out"=w311:string)  [unwired: 14 in]
      }
      frame "UI: Check Variants" {
        # "Do not put any code in this frame.\n(It is a separator no-op. You can make a copy of this frame to create a new UI frame)"
        n140 = Unbundle By Name(w319) -> ("Funnel Settings"=w321:refnum<class "Funnel Settings.lvclass">)
        n141 = property class="Funnel Settings.lvclass"(reference=w321) -> (reference out=w317:refnum<class "Funnel Settings.lvclass">, "Accessors:Speed Settings"=w316:variant, "Accessors:Voltage Settings"=w313:variant)  [unwired: 1 in, 1 out]
        n142 = call "Schedule.CheckVariantAttributes.vi"("error in (no error)"=w323, "Variant In"=w316) -> ("error out"=w325:errorcluster, "Variant Out"=w315:variant)  [unwired: 8 in]
        n143 = call "Schedule.CheckVariantAttributes.vi"("error in (no error)"=w325, "Variant In"=w313) -> ("error out"=w324:errorcluster, "Variant Out"=w314:variant)  [unwired: 8 in]
        n144 = property class="Funnel Settings.lvclass"(reference=w317, "Accessors:Speed Settings"=w315, "Accessors:Voltage Settings"=w314) -> (reference out=w318:refnum<class "Funnel Settings.lvclass">)  [unwired: 1 in, 1 out]
        n145 = Bundle By Name(cluster=w319, "Funnel Settings"=w318) -> (w320:T9)
        n146 = call <vilib>:"Add State(s) to Queue__JKI_lib_State_Machine.vi"("State(s) in (\"\")"=w327) -> ("States Out"=w326:string)  [unwired: 14 in]
      }
      frame "UI: Cursor Set" {
        # "Argument"
        # "Set and Unset Cursor Busy.\n(Usage: \"UI: Cursor Set >> Busy|Idle\")"
        n147 = case shown="\"Idle\", Default" w330 {
          tunnel: w332 -> [w336 w338]
          tunnel: [w335 w337] -> w331
          frame "Idle", Default {
            n148 = call <vilib>:"Unset Busy.vi"("error in (no error)"=w336) -> ("error out"=w335:errorcluster)  [unwired: 10 in]
          }
          frame "Busy" {
            n149 = call <vilib>:"Set Busy.vi"("error in (no error)"=w338) -> ("error out"=w337:errorcluster)  [unwired: 9 in, 1 out]
          }
        }
        n150 = call <vilib>:"Add State(s) to Queue__JKI_lib_State_Machine.vi"("State(s) in (\"\")"=w334) -> ("States Out"=w333:string)  [unwired: 14 in]
      }
      frame "UI: Update Speed/Voltage Visibility" {
        n151 = local read "Voltage Schedule"() -> (w347:u16)
        n152 = local read "Speed Schedule"() -> (w346:u16)
        n153 = case shown="0" w347 {
          tunnel: [TRUE FALSE] -> w349
          frame 0 {
          }
          frame 1, Default {
          }
        }
        n154 = case shown="0" w346 {
          tunnel: [TRUE FALSE] -> w348
          frame 0 {
          }
          frame 1, Default {
          }
        }
        n155 = property on="Voltage (V)" class="DigNum (strict)"(error in=w350, "Visible"=w349) -> (error out=w345:errorcluster)  [unwired: 1 in, 1 out]
        n156 = Not(x=w349) -> (.not. x?=w343:bool)
        n157 = property on="Voltage Settings" class="Bool (strict)"(error in=w345, "Visible"=w343) -> (error out=w344:errorcluster)  [unwired: 1 in, 1 out]
        n158 = property on="Speed (um/s)" class="DigNum (strict)"(error in=w344, "Visible"=w348) -> (error out=w342:errorcluster)  [unwired: 1 in, 1 out]
        n159 = Not(x=w348) -> (.not. x?=w341:bool)
        n160 = property on="Speed Settings" class="Bool (strict)"(error in=w342, "Visible"=w341) -> (error out=w340:errorcluster)  [unwired: 1 in, 1 out]
        n161 = call <vilib>:"Add State(s) to Queue__JKI_lib_State_Machine.vi"("State(s) in (\"\")"=w353) -> ("States Out"=w352:string)  [unwired: 14 in]
      }
      frame "UI: Front Panel State" {
        # "Argument"
        # "Set Front Panel Open or Closed\n(Usage: \"UI: Front Panel State >> Open|Close\")"
        n162 = Unbundle By Name(w359) -> ("Core.Current VI Reference"=w361:refnum<vi>)
        n163 = case shown="\"Open\", Default" w360 {
          tunnel: w363 -> [w369 w382]
          tunnel: [w371 w383] -> w362
          tunnel: w361 -> [w370 w380]
          frame "Open", Default {
            n164 = property class="VI"(reference=w370, error in=w369) -> (reference out=w367:refnum<vi>, error out=w368:errorcluster, "Front Panel.Open"=w366:bool)
            n165 = case shown="False" w366 {
              tunnel: [w374 w377] -> w371
              tunnel: w368 -> [w373 w377]
              tunnel: w367 -> [w372 _]
              frame False {
                n166 = invoke class="VI" method="FP.Open"(reference=w372, error in=w373, "Activate"=TRUE, "State"=T5."Standard") -> (error out=w374:errorcluster)  [unwired: 1 in, 4 out]
              }
              frame True {
              }
            }
          }
          frame "Close" {
            n167 = property class="VI"(reference=w380, error in=w382) -> (reference out=w379:refnum<vi>, error out=w381:errorcluster, "Front Panel.Open"=w378:bool)
            n168 = case shown="True" w378 {
              tunnel: [w384 w387] -> w383
              tunnel: w381 -> [w384 w386]
              tunnel: w379 -> [_ w385]
              frame False {
              }
              frame True {
                n169 = invoke class="VI" method="FP.Close"(reference=w385, error in=w386) -> (error out=w387:errorcluster)  [unwired: 1 in, 2 out]
              }
            }
          }
        }
        n170 = call <vilib>:"Add State(s) to Queue__JKI_lib_State_Machine.vi"("State(s) in (\"\")"=w365) -> ("States Out"=w364:string)  [unwired: 14 in]
      }
      frame "---------- Macro ----------" {
        # "Do not put any code in this frame.\n(It is a separator no-op. You can make a copy of this frame to create a new Macro frame)"
        n171 = call <vilib>:"Add State(s) to Queue__JKI_lib_State_Machine.vi"("State(s) in (\"\")"=w392) -> ("States Out"=w391:string)  [unwired: 14 in]
      }
      frame "Macro: Initialize" {
        # "Initialization Macro\n(This is called once, when the VI starts)"
        n172 = call <vilib>:"Add State(s) to Queue__JKI_lib_State_Machine.vi"("State(s) in Front (\"\")"="Data: Initialize\nInitialize Core Data\nDatabase: Locate\nEvents: Register\nUI: Initialize\n//UI: Check Variants\n//UI: Update Controls\n//UI: Update Speed/Voltage Visibility\nUI: Front Panel State >> Close", "State(s) in (\"\")"=w398) -> ("States Out"=w397:string)  [unwired: 13 in]
      }
      frame "Macro: Exit" {
        # "Exit Macro\n(This is called once, when the VI exits)"
        n173 = Unbundle By Name(w400) -> ("Core.Close Panel on Exit?"=w406:bool)
        n174 = Select(t="UI: Front Panel State >> Close", s=w406, f="") -> (s? t:f=w403:string)
        n175 = call <vilib>:"Add State(s) to Queue__JKI_lib_State_Machine.vi"("State(s) in (\"\")"=w403, "State(s) at Back (\"\")"="Data: Cleanup\nEvents: Unregister\nExit") -> ("States Out"=w401:string)  [unwired: 13 in]
        n176 = call <vilib>:"Add State(s) to Queue__JKI_lib_State_Machine.vi"("State(s) in Front (\"\")"=w401, "State(s) in (\"\")"=w409) -> ("States Out"=w408:string)  [unwired: 13 in]
      }
      frame "---------- Database ----------" {
        # "Template Separator\n(You can make a copy of, or modify, this frame)"
        n177 = call <vilib>:"Add State(s) to Queue__JKI_lib_State_Machine.vi"("State(s) in (\"\")"=w414) -> ("States Out"=w413:string)  [unwired: 14 in]
      }
      frame "Database: Set as Default" {
        # "Template Separator\n(You can make a copy of, or modify, this frame)"
        n178 = Unbundle By Name(w416) -> ("SettingDB"=w421:refnum<class "Setting Database.lvclass">)
        n179 = call "Setting Database.SetDefaultFunnel.vi"("error in (no error)"=w418, "SetDefaultFunnel"=T6 TRUE, "Setting Database"=w421) -> ("error out"=w419:errorcluster, "Setting Database out"=w415:refnum<class "Setting Database.lvclass">)  [unwired: 7 in]
        n180 = Bundle By Name(cluster=w416, "SettingDB"=w415) -> (w417:T9)
        n181 = call <vilib>:"Add State(s) to Queue__JKI_lib_State_Machine.vi"("State(s) in (\"\")"=w424) -> ("States Out"=w423:string)  [unwired: 14 in]
      }
      frame "Database: Copy to All" {
        # "Template Separator\n(You can make a copy of, or modify, this frame)"
        n182 = Unbundle By Name(w430) -> ("SettingDB"=w425:refnum<class "Setting Database.lvclass">)
        n183 = call "Setting Database.CopyActiveFunnelToAll.vi"("error in (no error)"=w427, "CopyActiveFunnelToAll"=T7 TRUE, "Setting Database"=w425) -> ("error out"=w426:errorcluster, "Setting Database out"=w429:refnum<class "Setting Database.lvclass">)  [unwired: 7 in]
        n184 = Bundle By Name(cluster=w430, "SettingDB"=w429) -> (w431:T9)
        n185 = call <vilib>:"Add State(s) to Queue__JKI_lib_State_Machine.vi"("State(s) in (\"\")"=w434) -> ("States Out"=w433:string)  [unwired: 14 in]
      }
      frame "Database: Locate" {
        w441 = refnum<class "Setting Database.lvclass"> refnum  # SettingDB
        # "#todo\nDecide what to do if not found..."
        # "Your code here.\n(You can make a copy of, or modify, this frame)"
        n186 = call <vilib>:"Create.vi"("SMO"=refnum<class "SMO.lvclass"> refnum) -> ("error out"=w446:errorcluster, "SMO out"=w448:refnum<class "SMO.lvclass">)  [unwired: 8 in, 1 out]
        n187 = call "Setting Database Name.vi"() -> ("Name"=w444:string)  [unwired: 10 in, 1 out]
        n188 = call <vilib>:"ListSharedResources.vi"("error in (no error)"=w446, "Filter (regex|name)"=w444, "SMO in"=w448) -> ("error out"=w445:errorcluster, "resources found?"=→"resources found?":bool, "Shared Resources"=w443:refnum<class "SMO.lvclass">[], "SMO out"=w447:refnum<class "SMO.lvclass">)  [unwired: 5 in]
        n189 = call <vilib>:"Destroy.vi"("error in (no error)"=w445, "SMO"=w447) -> ()  [unwired: 9 in, 1 out]
        n190 = Index Array(array=w443) -> (element=w442:refnum<class "SMO.lvclass">)  [unwired: 1 in]
        n191 = To More Specific Class(target class=w441, reference=w442) -> (specific class reference=w437:refnum<class "Setting Database.lvclass">)  [unwired: 1 in, 1 out]
        n192 = Bundle By Name(cluster=w438, "SettingDB"=w437) -> (w439:T9)
        n193 = call <vilib>:"Add State(s) to Queue__JKI_lib_State_Machine.vi"("State(s) in (\"\")"=w451) -> ("States Out"=w450:string)  [unwired: 14 in]
      }
      frame "Database: Update Active" {
        # "Your code here.\n(You can make a copy of, or modify, this frame)"
        n194 = Unbundle By Name(w457) -> ("SettingDB"=w456:refnum<class "Setting Database.lvclass">, "Funnel Settings"=w452:refnum<class "Funnel Settings.lvclass">)
        n195 = call "Setting Database.UpdateActiveFunnel.vi"("error in (no error)"=w453, "UpdateActiveFunnel"=w452, "Setting Database"=w456) -> ("error out"=w454:errorcluster, "Setting Database"=w455:refnum<class "Setting Database.lvclass">)  [unwired: 7 in]
        n196 = Bundle By Name(cluster=w457, "SettingDB"=w455) -> (w458:T9)
        n197 = call <vilib>:"Add State(s) to Queue__JKI_lib_State_Machine.vi"("State(s) in (\"\")"=w461) -> ("States Out"=w460:string)  [unwired: 14 in]
      }
    }
  }
